vi "(SUBVI) - Turn Left Degrees.vi"(8 "NXT/EV3":T1, 11 "Degrees":dbl) -> (0 "NXT/EV3 2":T1)   [LabVIEW 2016, in "testrobot.lvrbt"]
uses:
  testrobot.lvrbt
  <vilib>/NXT/Subs/LVHSConnector.ctl
  <vilib>/NXT/LegoClasses/BrickReference/BrickReference.lvclass
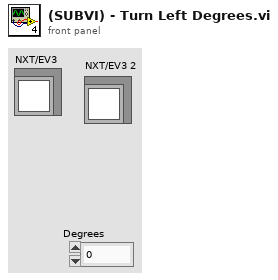
[diagram p1: front panel]
types:
  T1 = typedef "LVHSConnector.ctl" = refnum<class "BrickReference.lvclass">
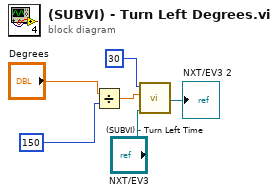
[diagram p0: block diagram]
diagram:
  n1 = Divide(x="Degrees", y=150) -> (x/y=w3:dbl)
  n2 = call "(SUBVI) - Turn Left Time.vi"("NXT/EV3"="NXT/EV3", "Time walking"=w3, "Walk Speed"=30) -> ("NXT/EV3 2"=→"NXT/EV3 2":T1)  [unwired: 8 in]
